vi "EPR measure gated new.vi"(9 "N loops":i32=-1, 10 "Measurement Interval":dbl=1.0, 11 "file path (dialog if empty)":path) -> ()   [LabVIEW 2012]
uses:
  <vilib>/DAQmx/read.llb/DAQmx Read (Counter U32 1Chan 1Samp).vi
  <vilib>/DAQmx/create/channels.llb/DAQmx Create Channel (CI-Count Edges).vi
  <vilib>/DAQmx/create/channels.llb/DAQmx Create Channel (CO-Pulse Generation-Ticks).vi
  <vilib>/DAQmx/configure/timing.llb/DAQmx Timing (Sample Clock).vi
  <vilib>/DAQmx/configure/timing.llb/DAQmx Timing (Implicit).vi
  <vilib>/Utility/file.llb/Write To Spreadsheet File (I64).vi
  <vilib>/DAQmx/miscellaneous.llb/DAQmx Fill In Error Info.vi
  <resource>/objmgr/daqmx.rc
panel:
  out "ref":u32
  in  "stop":bool
  out "signal":u32
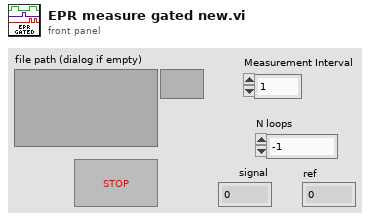
[diagram p1: front panel]
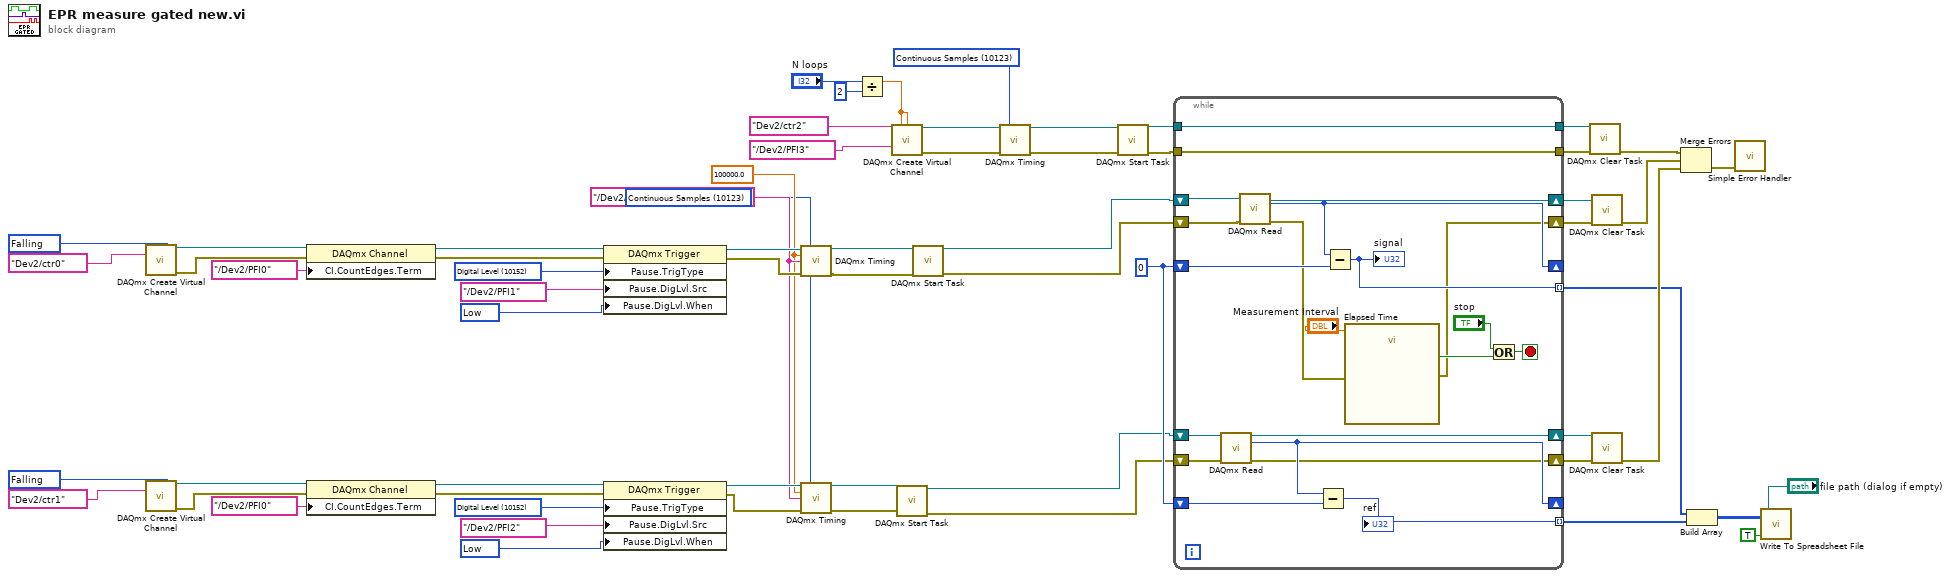
[diagram p0: block diagram]
diagram:
  w26 = 10214 items=["High"=10192, "Low"=10214] ("Pause.DigLvl.When")
  w28 = 10152 items=["Analog Level"=10101, "Analog Window"=10103, "Digital Level"=10152, "Digital Pattern"=10398, "None"=10230] ("Pause.TrigType")
  w29 = 10171 items=["Rising"=10280, "Falling"=10171] ("edge")
  w13 = u32 0 ("data")
  w32 = 10123 items=["Finite Samples"=10178, "Continuous Samples"=10123, "Hardware Timed Single Point"=12522] ("sample mode")
  w16 = tag "/Dev2/Ctr2InternalOutput" ("source")
  w14 = 10123 items=["Finite Samples"=10178, "Continuous Samples"=10123, "Hardware Timed Single Point"=12522] ("sample mode")
  w52 = 10214 items=["High"=10192, "Low"=10214] ("Pause.DigLvl.When")
  w54 = 10152 items=["Analog Level"=10101, "Analog Window"=10103, "Digital Level"=10152, "Digital Pattern"=10398, "None"=10230] ("Pause.TrigType")
  w55 = 10171 items=["Rising"=10280, "Falling"=10171] ("edge")
  w15 = 100000.0 ("rate")
  n1 = call-poly <vilib>:"DAQmx Create Virtual Channel.vi"("edge"=w29, "counter"=tag "Dev2/ctr0") -> ("task out"=w24:refnum<k21>, "error out"=w21:errorcluster)  [unwired: 7 in, 5 out]
  n2 = call-poly <vilib>:"DAQmx Create Virtual Channel.vi"("edge"=w55, "counter"=tag "Dev2/ctr1") -> ("task out"=w50:refnum<k21>, "error out"=w31:errorcluster)  [unwired: 7 in, 5 out]
  n3 = property class="DAQmx Channel"(reference=w24, error in=w21, "CI.CountEdges.Term"=tag "/Dev2/PFI0") -> (reference out=w25:refnum<k21>, error out=w23:errorcluster)
  n4 = property class="DAQmx Channel"(reference=w50, error in=w31, "CI.CountEdges.Term"=tag "/Dev2/PFI0") -> (reference out=w51:refnum<k21>, error out=w49:errorcluster)
  n5 = property class="DAQmx Trigger"(reference=w25, error in=w23, "Pause.TrigType"=w28, "Pause.DigLvl.Src"=tag "/Dev2/PFI1", "Pause.DigLvl.When"=w26) -> (reference out=w20:refnum<k21>, error out=w19:errorcluster)
  n6 = property class="DAQmx Trigger"(reference=w51, error in=w49, "Pause.TrigType"=w54, "Pause.DigLvl.Src"=tag "/Dev2/PFI2", "Pause.DigLvl.When"=w52) -> (reference out=w18:refnum<k21>, error out=w17:errorcluster)
  n7 = call-poly <vilib>:"DAQmx Timing.vi"("task/channels in"=w20, "sample mode"=w14, "rate"=w15, "source"=w16, "error in"=w19) -> ("task out"=w7:refnum<k21>, "error out"=w8:errorcluster)  [unwired: 9 in]
  n8 = call-poly <vilib>:"DAQmx Timing.vi"("task/channels in"=w18, "sample mode"=w14, "rate"=w15, "source"=w16, "error in"=w17) -> ("task out"=w6:refnum<k21>, "error out"=w5:errorcluster)  [unwired: 9 in]
  n9 = Divide(x="N loops", y=2) -> (x/y=w43:dbl)
  n10 = call-poly <vilib>:"DAQmx Create Virtual Channel.vi"("high ticks"=w43, "low ticks"=w43, "counter"=tag "Dev2/ctr2", "source of ticks"=tag "/Dev2/PFI3" ("source")) -> ("task out"=w41:refnum<k21>, "error out"=w34:errorcluster)  [unwired: 10 in]
  n11 = call <vilib>:"DAQmx Start Task.vi"("task/channels in"=w6, "error in"=w5) -> ("task out"=w4:refnum<k21>, "error out"=w3:errorcluster)  [unwired: 12 in]
  n12 = call <vilib>:"DAQmx Start Task.vi"("task/channels in"=w7, "error in"=w8) -> ("task out"=w2:refnum<k21>, "error out"=w1:errorcluster)  [unwired: 12 in]
  n13 = call-poly <vilib>:"DAQmx Timing.vi"("task/channels in"=w41, "sample mode"=w32, "error in"=w34) -> ("task out"=w35:refnum<k21>, "error out"=w33:errorcluster)  [unwired: 11 in]
  n14 = call <vilib>:"DAQmx Start Task.vi"("task/channels in"=w35, "error in"=w33) -> ("task out"=w40:refnum<k21>, "error out"=w39:errorcluster)  [unwired: 12 in]
  n15 = while {
    shift-right: [w73] -> w12
    shift-left: w2 -> [w84]
    tunnel: [w76] -> w47 mode=indexing
    tunnel: w40 -> [w80]
    tunnel: w39 -> [w79]
    tunnel: [w80] -> w38
    tunnel: [w79] -> w37
    shift-right: [w69] -> _
    shift-left: w13 -> [w78]
    shift-right: [w70] -> _
    shift-left: w13 -> [w77]
    shift-right: [w71] -> w61
    shift-left: w4 -> [w74]
    tunnel: [w68] -> w9 mode=indexing
    shift-right: [w67] -> w11
    shift-left: w1 -> [w64]
    shift-right: [w66] -> w10
    shift-left: w3 -> [w65]
    stop <- w83 stop-if-true
    n16 = call-poly <vilib>:"DAQmx Read.vi"("task/channels in"=w74, "error in"=w65) -> ("task out"=w71:refnum<k21>, "data"=w70:u32, "error out"=w66:errorcluster)  [unwired: 11 in]
    n17 = call-poly <vilib>:"DAQmx Read.vi"("task/channels in"=w84, "error in"=w64) -> ("task out"=w73:refnum<k21>, "data"=w69:u32, "error out"=w72:errorcluster)  [unwired: 11 in]
    n18 = Subtract(x=w70, y=w77) -> (x-y=w76:u32)
    "ref" <- w76
    n19 = Subtract(x=w69, y=w78) -> (x-y=w68:u32)
    "signal" <- w68
    n20 = call "Elapsed Time"("Time Target (s)"="Measurement Interval", "error in (no error)"=w72) -> ("Time has Elapsed"=w82:bool, "error out"=w67:errorcluster)  [unwired: 10 in, 6 out]
    n21 = Or(x="stop", y=w82) -> (x .or. y?=w83:bool)
  }
  n22 = call <vilib>:"DAQmx Clear Task.vi"("task in"=w38, "error in"=w37) -> ("error out"=w36:errorcluster)  [unwired: 13 in]
  n23 = call <vilib>:"DAQmx Clear Task.vi"("task in"=w12, "error in"=w11) -> ("error out"=w59:errorcluster)  [unwired: 13 in]
  n24 = call <vilib>:"DAQmx Clear Task.vi"("task in"=w61, "error in"=w10) -> ("error out"=w57:errorcluster)  [unwired: 13 in]
  n25 = Merge Errors(w36, w59, w57) -> (w58:errorcluster)
  n26 = Build Array(w9, w47) -> (w60:u32[][])
  n27 = call <vilib>:"Simple Error Handler.vi"("error in (no error)"=w58) -> ()  [unwired: 4 in, 5 out]
  n28 = call-poly <vilib>:"Write To Spreadsheet File.vi"("transpose? (no:F)"=TRUE, "2D data"=w60, "file path (dialog if empty)"="file path (dialog if empty)") -> ()  [unwired: 5 in, 1 out]
